vi "Update Plugins Data.vi"(8 "error in (no error)":errorcluster, 10 "Plugins":refnum<class "Plugin.lvclass">[](array[class]), 11 "Logging Thread in":refnum<class "Logging Thread.lvclass">) -> (0 "error out":errorcluster, 3 "Logging Thread out":refnum<class "Logging Thread.lvclass">)   [LabVIEW 2019, in "DSF Core.lvlib" / "Logging Thread.lvclass"]
uses:
  Logging Thread.lvclass
  Plugin/Plugin.lvclass
  Plugin Data.ctl
  Logging Thread.lvclass/Logging Thread.ctl
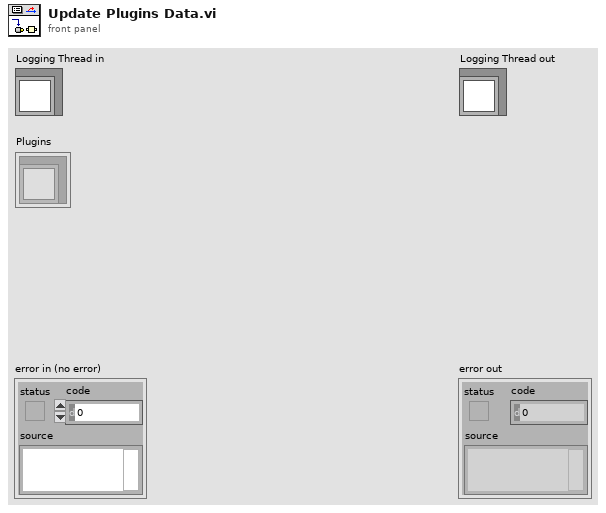
[diagram p1: front panel]
types:
  T1 = typedef "DSF Core.lvlib/Logging Thread.lvclass/Plugin Data.ctl" = cluster{"thread names":string[]}
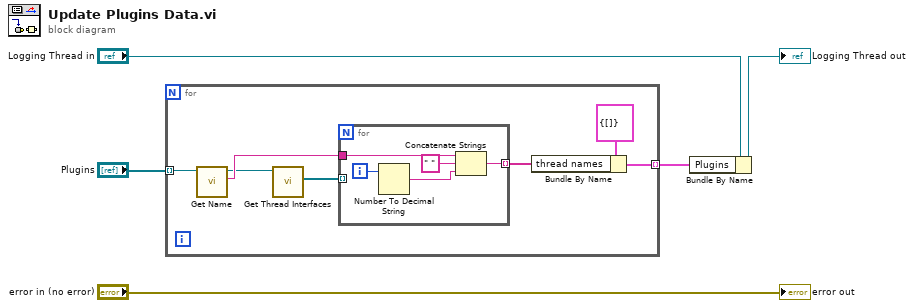
[diagram p0: block diagram]
diagram:
  n1 = for {
    tunnel: "Plugins" -> [w11] mode=indexing
    tunnel: [w10] -> w3 mode=indexing
    n2 = call "Get Name.vi"("Plugin in"=w11) -> ("name"=w9:string, "Plugin out"=w7:refnum<class "Plugin.lvclass">)  [unwired: 9 in]
    n3 = call "Get Thread Interfaces.vi"("Plugin in"=w7) -> ("Plugin Interfaces"=w6:refnum<class "Plugin Interface.lvclass">[])  [unwired: 9 in, 1 out]
    n4 = for {
      tunnel: w9 -> [w16]
      tunnel: [w15] -> w8 mode=indexing
      tunnel: w6 -> [_] mode=indexing
      i -> [w17]
      n5 = Number To Decimal String(number=w17) -> (decimal integer string=w14:string)  [unwired: 1 in]
      n6 = Concatenate Strings(w16, " " ("string"), w14) -> (w15:string)
    }
    n7 = Bundle By Name(cluster=T1 {"thread names"=[]} ("plugin data"), "thread names"=w8) -> (w10:T1)
  }
  n8 = Bundle By Name(cluster="Logging Thread in", "Plugins"=w3) -> (→"Logging Thread out":refnum<class "Logging Thread.lvclass">)
  "error out" <- "error in (no error)"
